vi "extract_depth_range_fix_width.vi"(4 "x offset":i32, 6 "width":i32=2, 7 "vertical offset":i32=2, 8 "error in (no error)":errorcluster, 9 "vertical size":i32=2, 10 "Image Dst":T1, 11 "Image":T1) -> (0 "error out":errorcluster, 2 "co-ordinates":i32[](array[numeric]), 3 "Image Dst Out":T1)   [LabVIEW 2016]
doc: "Extracts ROI from image with a specified 'width', off-centre by 'x offset' with top at y position 'vertical offset' and height 'vertical size'.\n\ns"
uses:
  <vilib>/vision/Image Controls.llb/IMAQ Image.ctl
  <vilib>/vision/NI_Vision_Development_Module.lvlib
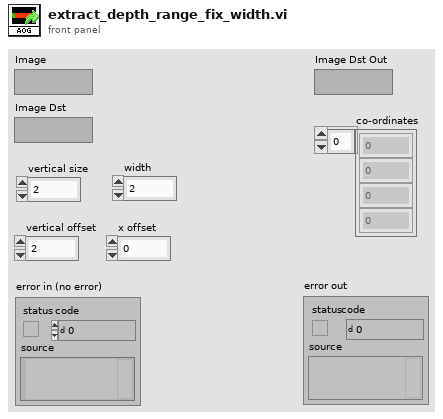
[diagram p1: front panel]
types:
  T1 = typedef "IMAQ Image.ctl" = refnum<image>
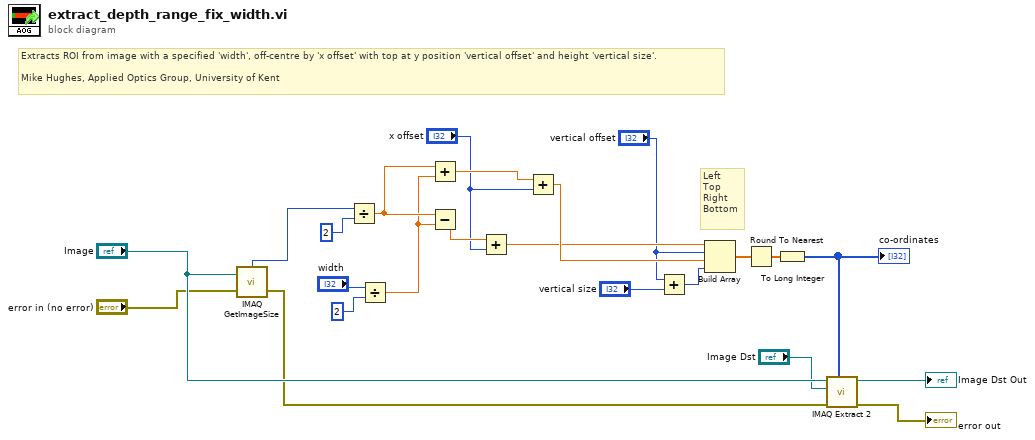
[diagram p0: block diagram]
diagram:
  # "Extracts ROI from image with a specified 'width', off-centre by 'x offset' with top at y position 'vertical offset' and height 'vertical size'.\n\nMike Hughes, Applied Optics Group, University of Kent"
  # "Left\nTop\nRight\nBottom"
  n1 = call "IMAQ GetImageSize"("Image"="Image", "error in (no error)"="error in (no error)") -> ("X Resolution"=w17:i32, "error out"=w18:errorcluster)  [unwired: 2 in, 1 out]
  n2 = Divide(x=w17, y=2) -> (x/y=w15:dbl)
  n3 = Divide(x="width", y=2) -> (x/y=w12:dbl)
  n4 = Add(x=w15, y=w12) -> (x+y=w11:dbl)
  n5 = Subtract(x=w15, y=w12) -> (x-y=w10:dbl)
  n6 = Add(x=w10, y="x offset") -> (x+y=w7:dbl)
  n7 = Add(x=w11, y="x offset") -> (x+y=w8:dbl)
  n8 = Add(x="vertical offset", y="vertical size") -> (x+y=w6:i32)
  n9 = Build Array(w7, "vertical offset", w8, w6) -> (w3:dbl[])
  n10 = Round To Nearest(number=w3) -> (nearest integer value=w2:dbl[])
  n11 = To Long Integer(number=w2) -> (32bit integer=w1:i32[])
  "co-ordinates" <- w1
  n12 = call "IMAQ Extract 2"("Optional Rectangle"=w1, "error in (no error)"=w18, "Image Dst"="Image Dst", "Image Src"="Image") -> ("error out"=→"error out":errorcluster, "Image Dst Out"=→"Image Dst Out":T1)  [unwired: 6 in]
